vi "VC840_RAW_Read.vi"(8 "error in (no error)":errorcluster, 11 "VISA resource name":refnum<visa-resource-name>) -> (0 "error out":errorcluster, 2 "Array":u8[](array[numeric]) format="%.0x", 3 "VISA resource name out":refnum<visa-resource-name>)   [LabVIEW 2013]
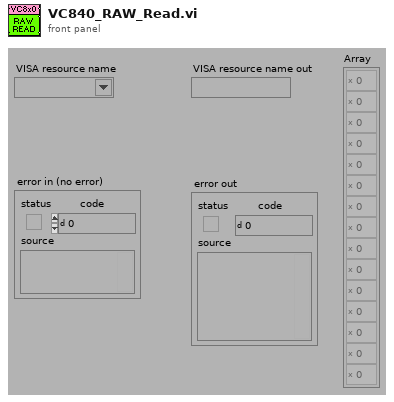
[diagram p1: front panel]
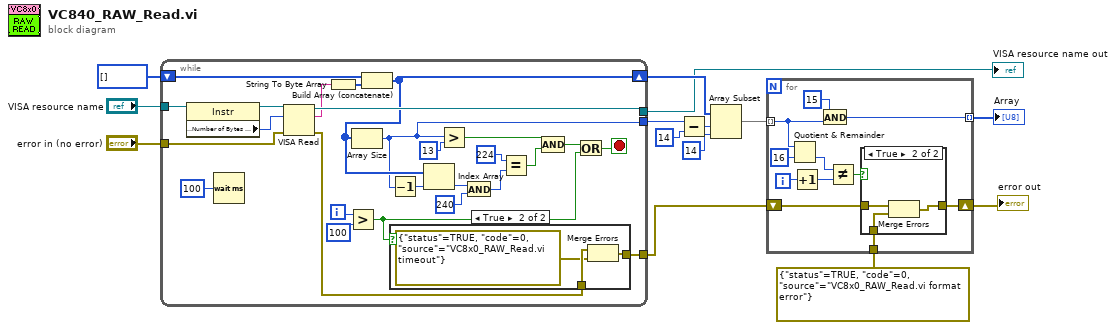
[diagram p0: block diagram]
diagram:
  n1 = while {
    tunnel: "error in (no error)" -> [w36]
    tunnel: "VISA resource name" -> [w38]
    tunnel: [w15] -> w14
    tunnel: [w35] -> w2
    shift-right: [w31] -> w6
    shift-left: u8[] [] -> [w34]
    tunnel: [w23] -> w11
    i -> [w20]
    stop <- w18 stop-if-true
    n2 = property class="Instr"(reference=w38) -> (reference out=w39:refnum<visa-resource-name>, "Serial Settings:Number of Bytes at Serial Port"=w37:u32)  [unwired: 1 in, 1 out]
    n3 = Wait (ms)(milliseconds to wait=u32 100) -> ()  [unwired: 1 out]
    n4 = VISA Read(VISA resource name=w39, byte count=w37, error in (no error)=w36) -> (VISA resource name out=w35:refnum<visa-resource-name>, read buffer=w21:string, error out=w16:errorcluster)  [unwired: 1 out]
    n5 = String To Byte Array(string=w21) -> (unsigned byte array=w33:u8[])
    n6 = Greater?(x=w20, y=100) -> (0:w17:bool)
    n7 = Build Array (concatenate)(w34, w33) -> (w31:u8[])
    n8 = Array Size(array=w31) -> (size(s)=w23:i32)
    n9 = Decrement(x=w23) -> (x-1=w22:i32)
    n10 = case shown="True" w17 {
      tunnel: w16 -> [w41 w44]
      tunnel: [w41 w43] -> w15
      frame False {
      }
      frame True {
        n11 = Merge Errors(w44, errorcluster {"status"=TRUE, "code"=0, "source"="VC8x0_RAW_Read.vi timeout"} ("error in 2 (no error)")) -> (w43:errorcluster)
      }
    }
    n12 = Index Array(array=w31, index=w22) -> (element=w30:u8)
    n13 = Greater?(x=w23, y=13) -> (0:w25:bool)
    n14 = And(x=w30, y=u8 240) -> (x .and. y?=w28:u8)
    n15 = Equal?(x=u8 224, y=w28) -> (x = y?=w26:bool)
    n16 = Compound Arithmetic op=AND(w25, w26) -> (w24:bool)
    n17 = Or(x=w24, y=w17) -> (x .or. y?=w18:bool)
  }
  "VISA resource name out" <- w2
  n18 = Subtract(x=w11, y=14) -> (x-y=w9:i32)
  n19 = Array Subset(array=w6, index=w9, length=14) -> (w5:u8[])
  n20 = for {
    tunnel: w5 -> [w54] mode=indexing
    shift-right: [w48] -> w3
    shift-left: w14 -> [w49]
    tunnel: [w46] -> w7 mode=indexing
    tunnel: errorcluster {"status"=TRUE, "code"=0, "source"="VC8x0_RAW_Read.vi format error"} ("error in 1 (no error)") -> [w45]
    i -> [w52]
    n21 = Quotient & Remainder(x=w54, y=u8 16) -> (floor(x/y)=w51:u8)  [unwired: 1 out]
    n22 = Increment(x=w52) -> (x+1=w50:i32)
    n23 = And(x=u8 15, y=w54) -> (x .and. y?=w46:u8)
    n24 = Not Equal?(x=w51, y=w50) -> (x != y?=w47:bool)
    n25 = case shown="True" w47 {
      tunnel: w49 -> [w56 w58]
      tunnel: [w56 w59] -> w48
      tunnel: w45 -> [_ w57]
      frame False {
      }
      frame True {
        n26 = Merge Errors(w58, w57) -> (w59:errorcluster)
      }
    }
  }
  "Array" <- w7
  "error out" <- w3
